vi "Process.vi"(8 "error in (no error)":errorcluster, 11 "RemoteControl":refnum<class "RemoteControl.lvclass">) -> (0 "error out":errorcluster, 3 "RemoteControl out":refnum<class "RemoteControl.lvclass">)   [LabVIEW 2019, in "RemoteControl.lvlib" / "RemoteControl.lvclass"]
doc: "---------------------------------------------------------------\nJKI State Machine Objects™\nhttp://jki.net/state-machine-objects/\nCopyright (C) 2005-2015, JKI <info@jki.net>\nALL RIGHTS RESERVED"
uses:
  RemoteControl.lvclass
  C:/Program Files/National Instruments/LabVIEW 2019/vi.lib/JKI/JKI SMO/SMO/SMO.lvclass
  RemoteControl.lvclass/RemoteControl.ctl
  Typedefs/Message--Cluster.ctl
  <vilib>/JKI/JKI SMO/SMO/Typedefs/Public Events.ctl
  <vilib>/JKI/JKI SMO/SMO/Typedefs/SMOState --Enum.ctl
  <vilib>/JKI/JKI SMO/SMO/Typedefs/Reserve State--Enum.ctl
  <vilib>/JKI/JKI SMO/SMO/SMO.lvclass/SMO.ctl
  Typedefs/RC Process Type--Enum.ctl
  <vilib>/JKI/JKI SMO/SMO/Private/ReftoDVR--SMO.vi
  <vilib>/dlg_ctls.llb/Space Constant.vi
  <vilib>/AdvancedString/1D String Array to Delimited String.vi
  <vilib>/JKI/JKI SMO/SMO/SMO.lvclass
  <userlib>/LevyLab/Debug/Debug.lvlib
panel:
  in  "create message error":bool
  out "Process Type":string
  out "Message Out":string
  out "Message In":string
  in  "delay response":bool
  in  "create server error":bool
  in  "create listener error":bool
  out "State History":string
  out "Connections":i32
  in  "Message Timing?":bool
  in  "timeout (ms)":i32=500
  in  "stop":bool
  # "Remote Control"
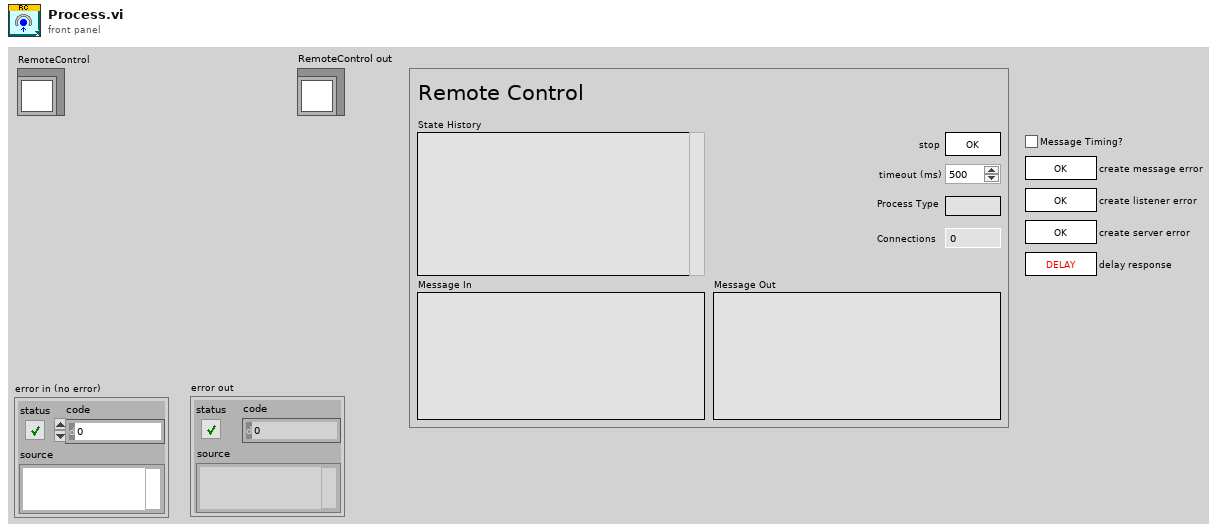
[diagram p1: front panel]
types:
  T1 = enum32{"invalid app kind", "Development System", "Run Time System", "Student Edition", "Embedded LabVIEW", "Evaluation", "Custom"}
  T2 = enum32{"Invalid", "Standard", "Closed", "Hidden", "Minimized", "Maximized"}
  T3 = typedef "RemoteControl.lvlib/RemoteControl.lvclass/Message--Cluster.ctl" = cluster{"Command":string, "Data":variant, "ID":string, "error":errorcluster}
  T4 = typedef "RemoteControl.lvlib/RemoteControl.lvclass/RC Process Type--Enum.ctl" = enum16{"Listener", "Server", "Client"}
  T5 = typedef "RemoteControl.lvlib/RemoteControl.lvclass/PrivateEvents--RemoteControl.Configure.ctl" = cluster{"address":string, "Port":u16, "AllowedRemote":string, "Commands":string[], "timeout":i32}
  T6 = cluster{"Core":cluster{"Current VI Reference":refnum<vi>, "Close Panel on Exit?":bool, "Last Error":cluster{"error":errorcluster, "previous state":string, "remaining states":string}, "Shutdown?":bool}, "SMO":refnum<class "RemoteControl.lvclass">, "Listener":refnum<class "RemoteControl.lvclass">, "RC Process Type":T4, "Configure":T5, "Messages (in)":T3[], "Messages (out)":T3[], "state":enum16{"waiting", "processing"}, "to":i32}
  T7 = cluster{"Current VI Reference":refnum<vi>, "Close Panel on Exit?":bool, "Last Error":cluster{"error":errorcluster, "previous state":string, "remaining states":string}, "Shutdown?":bool}
  T8 = typedef "Debug.lvlib/Attribute.Debug.lvclass/DebugBehavior.ctl" = enum16{"Normal", "Debug"}
  T9 = typedef "SMO.lvclass/Public Events.ctl" = cluster{"Error":refnum<user-event>, "State":refnum<user-event>, "Reserve State":refnum<user-event>}
  T10 = typedef "SMO.lvclass/Protected Events.ctl" = cluster{"StopProcesses":refnum<user-event>, "AbortProcesses":refnum<user-event>, "Config Changed":refnum<user-event>, "Dependency":refnum<user-event>}
  T11 = typedef "RemoteControl.lvlib/RemoteControl.lvclass/PrivateEvents--Cluster.ctl" = cluster{"Configure":refnum<user-event>, "SendMessageToProcess":refnum<user-event>}
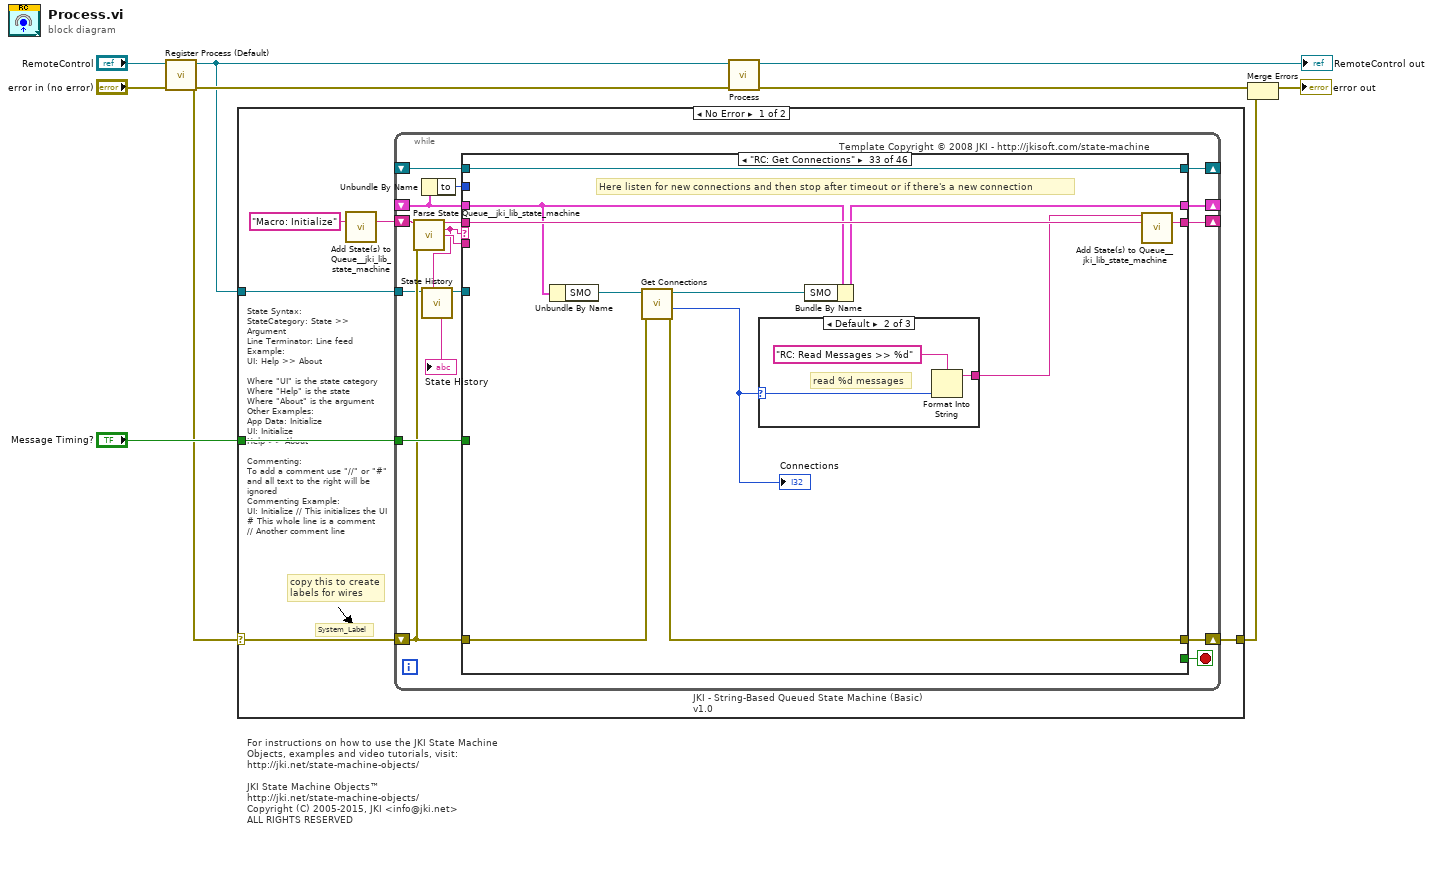
[diagram p0: block diagram]
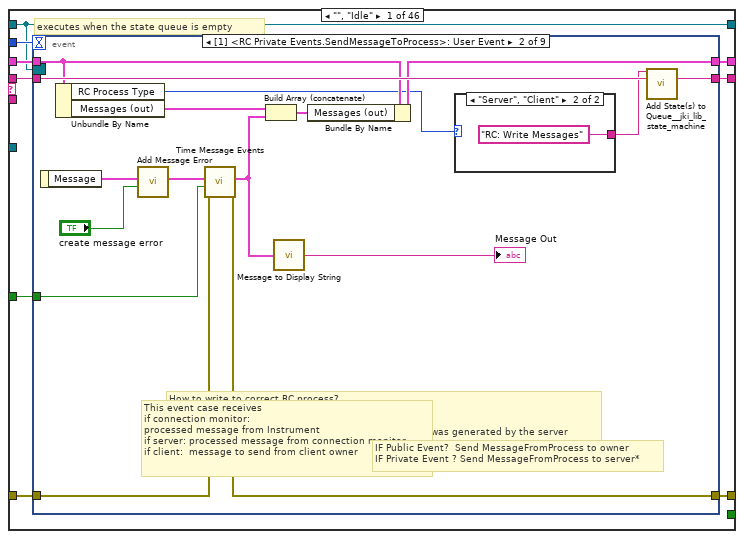
[diagram p2: hidden frame]
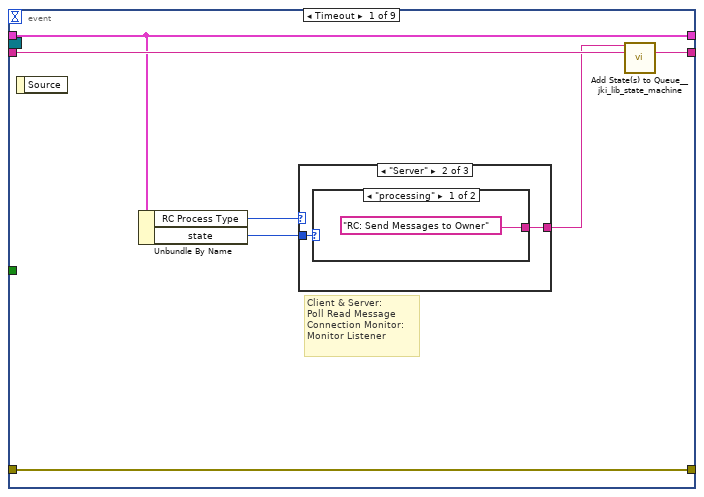
[diagram p3: hidden frame]
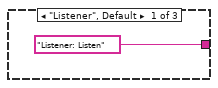
[diagram p4: hidden frame]
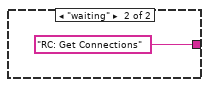
[diagram p5: hidden frame]
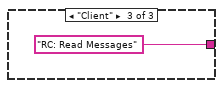
[diagram p6: hidden frame]
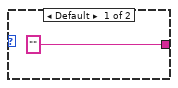
[diagram p7: hidden frame]
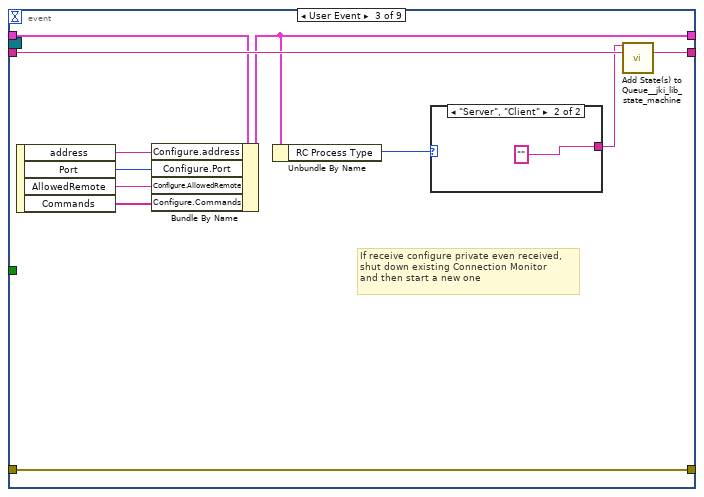
[diagram p8: hidden frame]
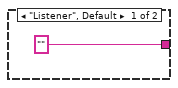
[diagram p9: hidden frame]
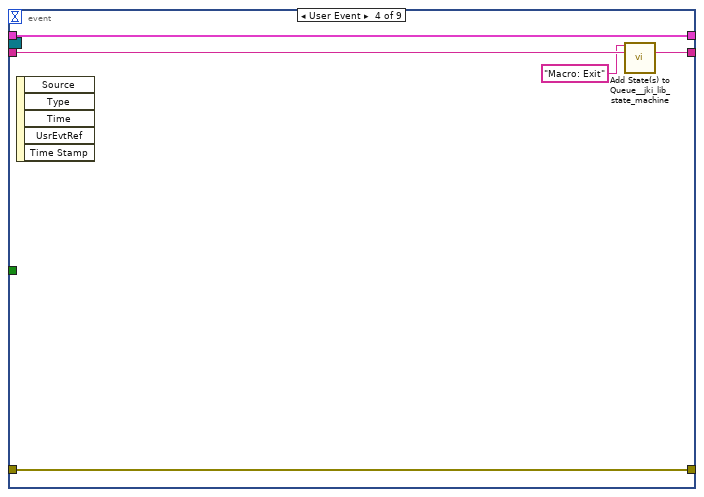
[diagram p10: hidden frame]
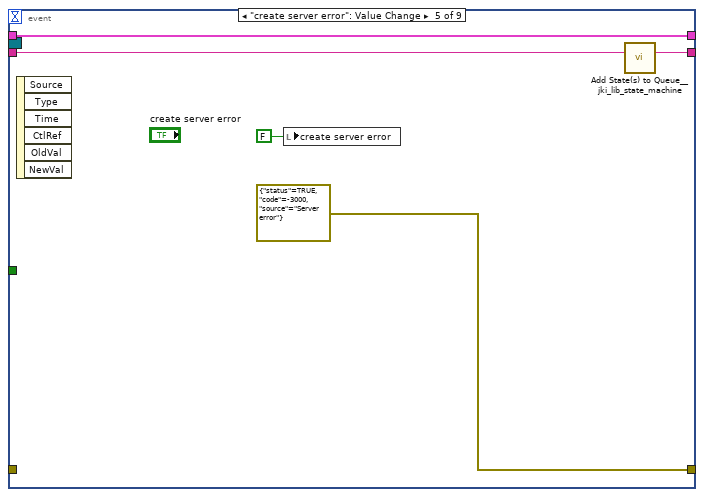
[diagram p11: hidden frame]
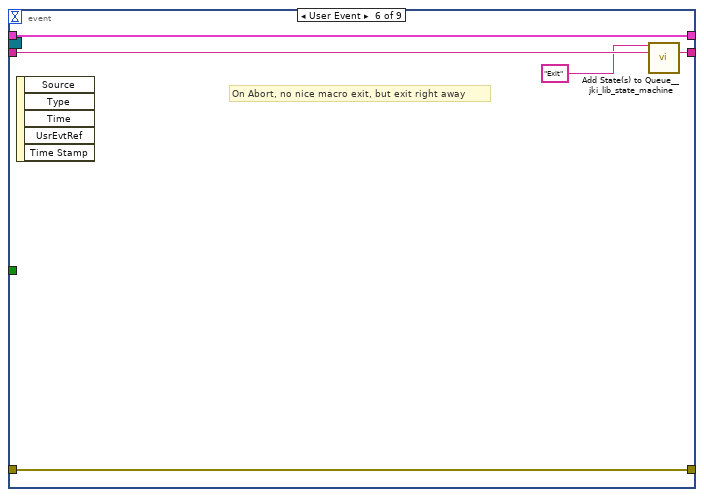
[diagram p12: hidden frame]
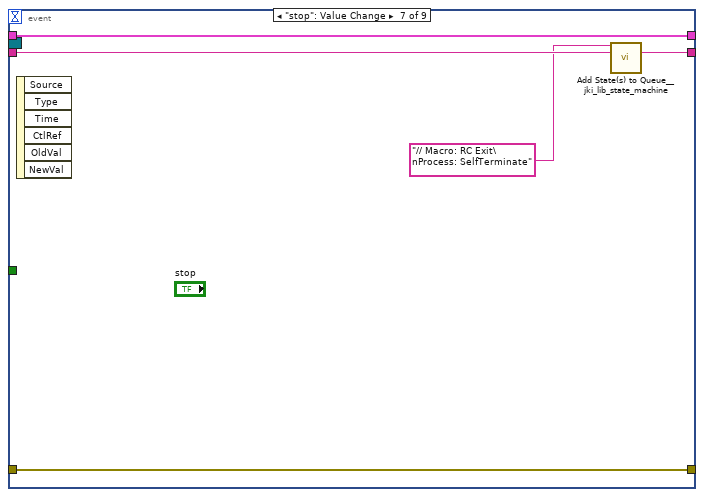
[diagram p13: hidden frame]
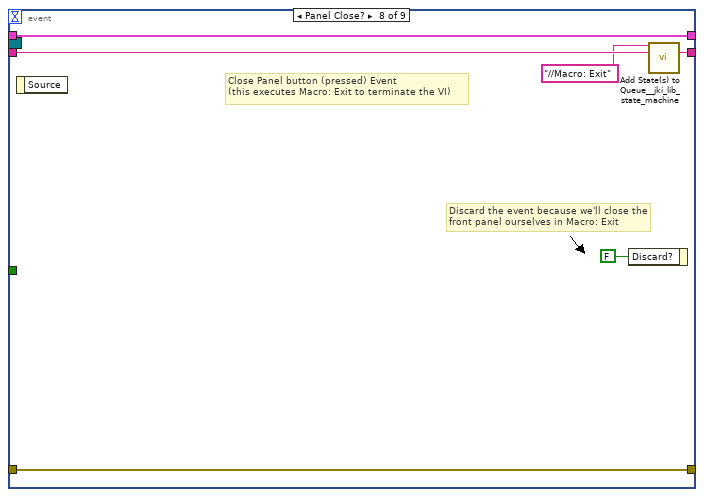
[diagram p14: hidden frame]
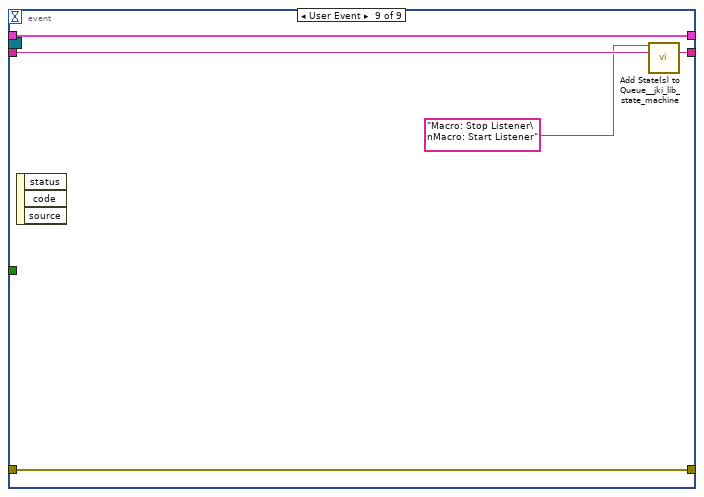
[diagram p15: hidden frame]
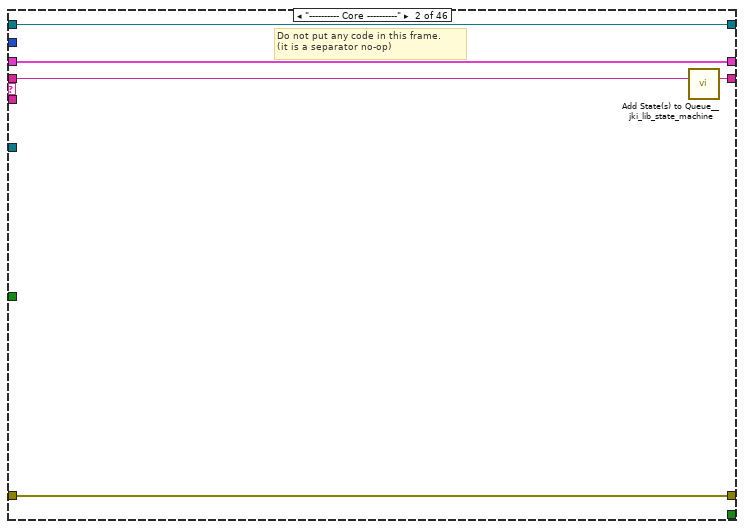
[diagram p16: hidden frame]
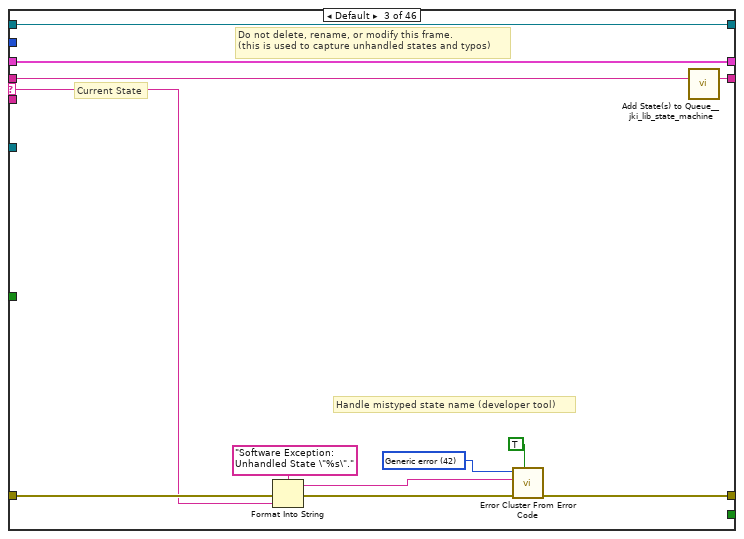
[diagram p17: hidden frame]
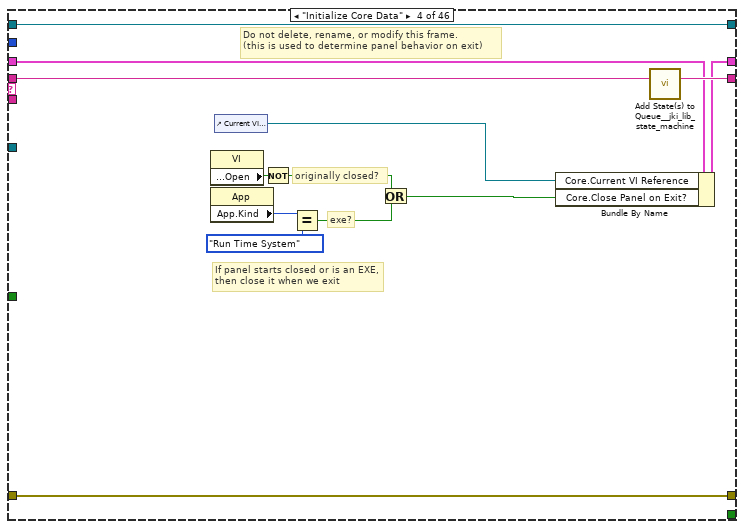
[diagram p18: hidden frame]
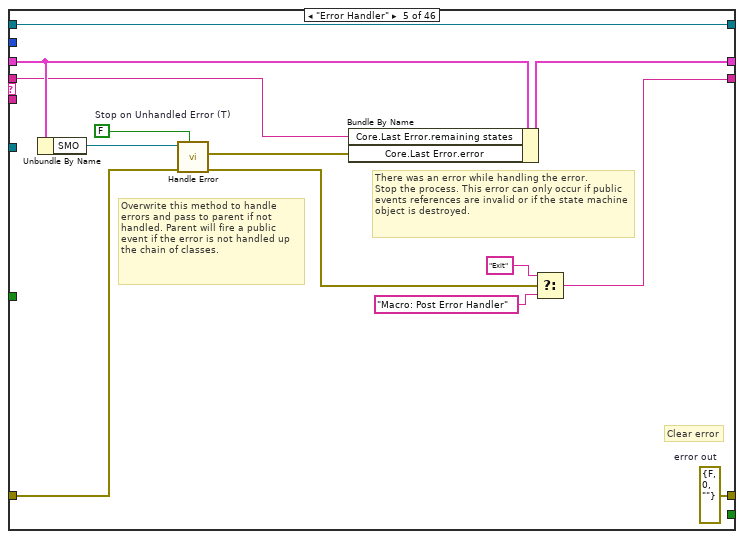
[diagram p19: hidden frame]
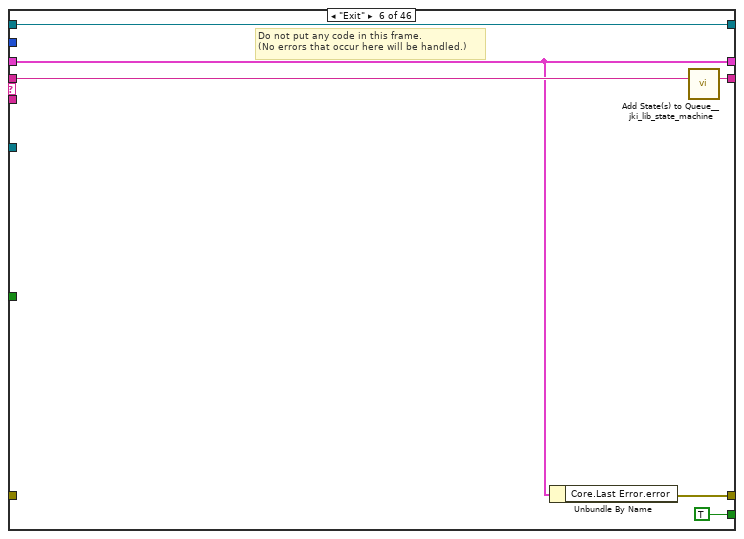
[diagram p20: hidden frame]
diagram:
  # "For instructions on how to use the JKI State Machine Objects, examples and video tutorials, visit:\nhttp://jki.net/state-machine-objects/\n\nJKI State Machine Objects™\nhttp://jki.net/state-machine-objects/\nCopyright (C) 2005-2015, JKI <info@jki.net>\nALL RIGHTS RESERVED"
  n1 = call <vilib>:"Register Process (Default).vi"("error in (no error)"="error in (no error)", "SMO"="RemoteControl") -> ("error out"=w3:errorcluster, "SelfRef"=w2:refnum<class "RemoteControl.lvclass">)  [unwired: 8 in]
  n2 = case shown="No Error" w3 {
    selector: w3 -> [w12 w656]
    tunnel: w2 -> [w13 _]
    tunnel: [w11 w656] -> w5
    tunnel: "Message Timing?" -> [w10 _]
    frame No Error {
      # "State Syntax:\nStateCategory: State >> Argument\nLine Terminator: Line feed\nExample:\nUI: Help >> About\n\nWhere \"UI\" is the state category\nWhere \"Help\" is the state\nWhere \"About\" is the argument\nOther Examples:\nApp Data: Initialize\nUI: Initialize\nHelp >> About\n\nCommenting:\nTo add a comment use \"//\" or \"#\" and all text to the right will be ignored\nCommenting Example:\nUI: Initialize // This initializes the UI\n# This whole line is a comment\n// Another comment line"
      # "copy this to create labels for wires"
      # "System_Label"
      n3 = call <vilib>:"Add State(s) to Queue__jki_lib_state_machine.vi"("State(s) in (\"\")"="Macro: Initialize") -> ("States Out"=w15:string)  [unwired: 14 in]
      n4 = while "JKI - String-Based Queued State Machine (Basic) v1.0" {
        shift-right: [w27] -> _
        shift-left: _ -> [w20]
        shift-right: [w29] -> w11
        shift-left: w12 -> [w23]
        shift-right: [w21] -> _
        shift-left: w15 -> [w30]
        tunnel: w13 -> [w16]
        shift-right: [w26] -> _
        shift-left: _ -> [w25]
        tunnel: w10 -> [w24]
        stop <- w28 stop-if-true
        # "Template Copyright © 2008 JKI - http://jkisoft.com/state-machine"
        n5 = call <vilib>:"Parse State Queue__jki_lib_state_machine.vi"("State Queue"=w30, "Error In (no error)"=w23) -> ("Remaining States"=w32:string, "Current State"=w22:string, "Arguments"=w31:string)  [unwired: 11 in]
        n6 = Unbundle By Name(w20) -> ("to"=w19:i32)
        n7 = call <userlib>:"State History.vi"("Current State"=w22, "SMO"=w16) -> ("SMO"=w17:refnum<class "RemoteControl.lvclass">, "History"=→"State History":string)  [unwired: 8 in]
        n8 = case shown="\"RC: Get Connections\"" w22 {
          selector: w22 -> [_ _ w123 _ _ _ _ _ _ _ _ _ _ _ _ _ _ _ _ _ _ _ _ _ _ _ _ _ _ _ _ _ _ _ _ _ _ _ _ _ _ _ _ _ _ _]
          tunnel: w32 -> [w41 w121 w127 w146 w149 w165 w170 w185 w192 w197 w207 w218 w234 w269 w274 w286 w301 w314 w326 w337 w346 w363 w385 w390 w401 w410 w415 w429 w443 w449 w454 w463 w482 w509 w538 w559 w572 w581 w590 w597 w608 w619 w624 w633 w645 w655]
          tunnel: w31 -> [_ _ _ _ _ _ _ _ _ _ _ w212 w229 w263 _ _ _ _ _ _ _ _ _ _ _ _ _ _ _ _ _ _ _ _ _ _ _ _ _ _ _ _ _ _ _ _]
          tunnel: [w38 w119 w129 w143 w158 w160 w168 w177 w189 w195 w199 w213 w227 w264 w272 w284 w292 w310 w318 w329 w344 w361 w383 w388 w393 w403 w413 w423 w438 w445 w450 w460 w472 w502 w531 w551 w567 w573 w582 w591 w603 w614 w620 w628 w634 w650] -> w29
          tunnel: [w40 w120 w126 w145 w152 w164 w169 w184 w191 w196 w206 w217 w233 w268 w273 w285 w300 w313 w325 w336 w345 w362 w384 w389 w400 w409 w414 w428 w442 w448 w453 w462 w481 w508 w537 w558 w571 w580 w589 w596 w607 w618 w623 w632 w644 w654] -> w21
          tunnel: [_ _ _ _ _ TRUE _ _ _ _ _ _ _ _ _ _ _ _ _ _ _ _ _ _ _ _ _ _ _ _ _ _ _ _ _ _ _ _ _ _ _ _ _ _ _ _] -> w28
          tunnel: [w36 w118 w125 w144 w156 w161 w167 w181 w188 w194 w204 w216 w231 w266 w271 w276 w290 w308 w322 w333 w341 w359 w374 w387 w398 w407 w412 w427 w441 w447 w452 w455 w479 w505 w529 w554 w568 w577 w584 w592 w600 w612 w622 w626 w641 w649] -> w27
          tunnel: w19 -> [w35 _ _ _ _ _ _ _ _ _ _ _ _ _ _ _ _ _ _ _ _ _ _ _ _ _ _ _ _ _ _ _ _ _ _ _ _ _ _ _ _ _ _ _ _ _]
          tunnel: w17 -> [_ _ _ _ _ _ _ w173 _ _ _ _ _ _ _ _ _ _ _ _ _ _ _ _ _ _ _ _ _ _ _ _ _ _ _ _ _ _ _ _ _ _ _ _ _ _]
          tunnel: [w34 w117 w122 w134 w159 w162 w166 w183 w187 w193 w205 w215 w228 w267 w270 w283 w299 w312 w324 w335 w343 w360 w379 w386 w399 w408 w411 w426 w440 w446 w451 w461 w480 w507 w536 w557 w570 w579 w588 w595 w606 w617 w621 w631 w643 w653] -> w26
          tunnel: w25 -> [w34 w117 w122 w134 w159 w162 w166 w183 w187 w193 w205 w215 w228 w267 w270 w283 w299 w312 w324 w335 w343 w360 w379 w386 w399 w408 w411 _ w436 w446 w451 w461 w480 w507 w536 w557 w570 w579 w588 w595 w606 w617 w621 w631 w643 w653]
          tunnel: w24 -> [w33 _ _ _ _ _ _ _ _ _ _ _ _ _ _ _ _ _ _ _ _ _ _ _ _ _ _ _ _ _ _ w458 _ w506 w534 _ _ _ _ _ _ _ _ _ _ _]
          tunnel: w23 -> [w37 w119 w128 w143 w154 _ w168 w177 w190 w195 w198 w214 w232 w265 w272 w284 w291 w310 w319 w330 w344 w361 w383 w388 w394 w404 w413 w424 w439 w445 w450 w457 w476 w495 w532 w552 w560 w574 w583 w594 w604 w615 w620 w629 w638 w651]
          tunnel: w20 -> [w39 w118 w125 w137 w157 w161 w167 _ w188 w194 w204 w216 w231 w266 w271 w276 w289 w308 w322 w333 w341 w356 w373 w387 w398 w402 w412 w427 w441 w447 w452 w455 w478 w497 w530 w555 w569 w578 w585 w592 w601 w609 w622 w625 w642 w649]
          frame "", "Idle" {
            # "executes when the state queue is empty"
            n9 = event shown="[1] <RC Private Events.SendMessageToProcess>: User Event" {
              selector: w34 -> [_ _ _ _ _ _ _ _ _]
              dyn-events: _ -> [_ _ _ _ _ _ _ _ _]
              timeout: w35 -> [_ _ _ _ _ _ _ _ _]
              tunnel: w41 -> [w48 w70 w82 w90 w95 w100 w104 w111 w116]
              tunnel: [w47 w69 w81 w89 w94 w99 w105 w110 w115] -> w40
              tunnel: w39 -> [w43 w66 w80 w87 w93 w97 w103 w108 w113]
              tunnel: [w46 w63 w83 w88 errorcluster {"status"=TRUE, "code"=-3000, "source"="Server error"} ("t") w98 w101 w109 w114] -> w38
              tunnel: w37 -> [w46 w62 w83 w88 _ w98 w101 w109 w114]
              tunnel: [w43 w68 w78 w87 w93 w97 w103 w108 w113] -> w36
              tunnel: w33 -> [_ w58 _ _ _ _ _ _ _]
              event Timeout {
                # "Client & Server:\nPoll Read Message\nConnection Monitor:\nMonitor Listener"
                n10 = event-data() -> ()  [unwired: 1 in, 1 out]
                n11 = Unbundle By Name(w43) -> ("RC Process Type"=w44:T4, "state"=w42:enum16{"waiting", "processing"})
                n12 = case shown="\"Server\"" w44 {
                  tunnel: ["Listener: Listen" ("State(s) in Front (\"\")") w51 "RC: Read Messages" ("State(s) in Front (\"\")")] -> w45
                  tunnel: w42 -> [_ w50 _]
                  frame "Listener", Default {
                  }
                  frame "Server" {
                    n13 = case shown="\"processing\"" w50 {
                      tunnel: ["RC: Send Messages to Owner" ("State(s) in Front (\"\")") "RC: Get Connections" ("State(s) in Front (\"\")")] -> w51
                      frame "processing" {
                      }
                      frame "waiting" {
                      }
                    }
                  }
                  frame "Client" {
                  }
                }
                n14 = call <vilib>:"Add State(s) to Queue__jki_lib_state_machine.vi"("State(s) in Front (\"\")"=w45, "State(s) in (\"\")"=w48) -> ("States Out"=w47:string)  [unwired: 13 in]
              }
              event User Event {
                # "IF Public Event?  Send MessageFromProcess to owner\nIF Private Event ? Send MessageFromProcess to server*"
                # "How to write to correct RC process?\nsomehow keep track of elements in\nserver SMO array\nMessage ID was generated when original public event was generated by the server"
                # "This event case receives\nif connection monitor:\nprocessed message from Instrument\nif server: processed message from connection monitor\nif client:  message to send from client owner"
                n15 = event-data() -> ("Message"=w57:T3)  [unwired: 1 in]
                n16 = Unbundle By Name(w66) -> ("RC Process Type"=w61:T4, "Messages (out)"=w65:T3[])
                n17 = call "Add Message Error.vi"("create message error"="create message error", "Message in"=w57) -> ("Message out"=w56:T3)  [unwired: 9 in]
                n18 = call "Time Message Events.vi"("error in (no error)"=w62, "Debug Mode"=w58, "Message in"=w56) -> ("error out"=w63:errorcluster, "Message out"=w59:T3)  [unwired: 5 in, 2 out]
                n19 = Build Array (concatenate)(w65, w59) -> (w64:T3[])
                n20 = call "Message to Display String.vi"("Message"=w59) -> ("message string"=→"Message Out":string)
                n21 = Bundle By Name(cluster=w66, "Messages (out)"=w64) -> (w68:T6)
                n22 = case shown="\"Server\", \"Client\"" w61 {
                  tunnel: ["" ("State(s) in Front (\"\")") "RC: Write Messages" ("State(s) in Front (\"\")")] -> w67
                  frame Default {
                  }
                  frame "Server", "Client" {
                  }
                }
                n23 = call <vilib>:"Add State(s) to Queue__jki_lib_state_machine.vi"("State(s) in Front (\"\")"=w67, "State(s) in (\"\")"=w70) -> ("States Out"=w69:string)  [unwired: 13 in]
              }
              event User Event {
                # "If receive configure private even received,\nshut down existing Connection Monitor \nand then start a new one"
                n24 = event-data() -> ("address"=w73:string, "Port"=w74:u16, "AllowedRemote"=w75:string, "Commands"=w76:string[])  [unwired: 1 in]
                n25 = Bundle By Name(cluster=w80, "Configure.address"=w73, "Configure.Port"=w74, "Configure.AllowedRemote"=w75, "Configure.Commands"=w76) -> (w78:T6)
                n26 = Unbundle By Name(w78) -> ("RC Process Type"=w79:T4)
                n27 = case shown="\"Server\", \"Client\"" w79 {
                  tunnel: ["" ("State(s) in Front (\"\")") "" ("State(s) in Front (\"\")")] -> w77
                  frame "Listener", Default {
                  }
                  frame "Server", "Client" {
                  }
                }
                n28 = call <vilib>:"Add State(s) to Queue__jki_lib_state_machine.vi"("State(s) in Front (\"\")"=w77, "State(s) in (\"\")"=w82) -> ("States Out"=w81:string)  [unwired: 13 in]
              }
              event User Event {
                n29 = event-data() -> ()  [unwired: 1 in, 5 out]
                n30 = call <vilib>:"Add State(s) to Queue__jki_lib_state_machine.vi"("State(s) in Front (\"\")"="Macro: Exit", "State(s) in (\"\")"=w90) -> ("States Out"=w89:string)  [unwired: 13 in]
              }
              event "create server error": Value Change {
                n31 = event-data() -> ()  [unwired: 1 in, 6 out]
                n32 = local write "create server error"(FALSE ("create listener error")) -> ()
                n33 = call <vilib>:"Add State(s) to Queue__jki_lib_state_machine.vi"("State(s) in (\"\")"=w95) -> ("States Out"=w94:string)  [unwired: 14 in]
              }
              event User Event {
                # "On Abort, no nice macro exit, but exit right away"
                n34 = event-data() -> ()  [unwired: 1 in, 5 out]
                n35 = call <vilib>:"Add State(s) to Queue__jki_lib_state_machine.vi"("State(s) in Front (\"\")"="Exit", "State(s) in (\"\")"=w100) -> ("States Out"=w99:string)  [unwired: 13 in]
              }
              event "stop": Value Change {
                n36 = event-data() -> ()  [unwired: 1 in, 6 out]
                n37 = call <vilib>:"Add State(s) to Queue__jki_lib_state_machine.vi"("State(s) in Front (\"\")"="// Macro: RC Exit\nProcess: SelfTerminate" ("State(s) in Front (\"\")"), "State(s) in (\"\")"=w104) -> ("States Out"=w105:string)  [unwired: 13 in]
              }
              event Panel Close? {
                # "Discard the event because we'll close the front panel ourselves in Macro: Exit"
                # "Close Panel button (pressed) Event\n(this executes Macro: Exit to terminate the VI)"
                n38 = event-data() -> ()  [unwired: 1 in, 1 out]
                n39 = event-data("Discard?"=FALSE) -> ()  [unwired: 1 in, 1 out]
                n40 = call <vilib>:"Add State(s) to Queue__jki_lib_state_machine.vi"("State(s) in Front (\"\")"="//Macro: Exit", "State(s) in (\"\")"=w111) -> ("States Out"=w110:string)  [unwired: 13 in]
              }
              event User Event {
                n41 = event-data() -> ()  [unwired: 1 in, 3 out]
                n42 = call <vilib>:"Add State(s) to Queue__jki_lib_state_machine.vi"("State(s) in Front (\"\")"="Macro: Stop Listener\nMacro: Start Listener", "State(s) in (\"\")"=w116) -> ("States Out"=w115:string)  [unwired: 13 in]
              }
            }
          }
          frame "---------- Core ----------" {
            # "Do not put any code in this frame.\n(it is a separator no-op)"
            n43 = call <vilib>:"Add State(s) to Queue__jki_lib_state_machine.vi"("State(s) in (\"\")"=w121) -> ("States Out"=w120:string)  [unwired: 14 in]
          }
          frame Default {
            w132 = 42 items=["No error", "Argument error", "Memory is full", "Out of zone", "End of file", "File already open", "Generic file I/O error", "File not found", "File permission error", "Disk is full", "Duplicate path", "Too many files open", "System feature not enabled", "Resource file not found", "Cannot add resource", "Resource not found", "Image not found", "Image memory error", "Pen does not exist", "Config type invalid", "Config token not found", "Config parse error", "Config memory error", "Bad external code format", "Bad external code offset", "External code not present", "Null window", "Destroy window error", "Null menu", "Print aborted", "Bad print record", "Print driver error", "Windows error during printing", "Memory error during printing", "Print dialog error", "Generic print error", "Invalid device refnum", "Device not found", "Device parameter error", "Device unit error", "Cannot open device", "Device call aborted", "Generic error", "Cancelled by user", "Object ID too low", "Object ID too high", "Object not in heap", "Unknown heap", "Unknown object (invalid DefProc)", "Unknown object (DefProc not in table)", "Message out of range", "Invalid (null) method", "Unknown message", "Manager call not supported", "Bad address", "Network operation in progress", "Network operation timed out", "Connection is busy", "Network attribute not supported", "Network error", "Address in use", "System out of memory", "Connection aborted", "Connection refused", "Not connected", "Already connected", "Connection closed", "Initialization error (interapplication manager)", "Bad occurrence", "Wait on unbound occurrence handler", "Occurrence queue overflow", "Datalog type conflict", "Unused", "Unrecognized type (interapplication manager)", "Memory corrupt", "Failed to make temporary DLL", "Old CIN version", "Drag socket not found", "Failed to load drop-object", "Failed to register OLE object", "Failed to release OLE object", "Format specifier type mismatch", "Unknown format specifier", "Too few format specifiers", "Too many format specifiers", "Scan failed", "Newer CIN version", "Error converting to variant", "Runtime menu error", "Password tampered", "Variant attribute not found", "Incompatible variant data type", "Event data is not available", "Event Store is not present", "Occurrence is not found", "Event Queue is not created", "Event info is not available", "Refnum passed is NULL", "Error retrieving Class GUID", "Error retrieving CoClass GUID", "Error retrieving TypeLib GUID.", "Bad built application magic bytes.", "Specific driver is different from the specific driver associated with the Logical Name.", "There is no session opened to the class driver.", "Max Error", "MAX - Error with config objects", "MAX - Error loading configuration", "MAX - Group not supported"]
            # "Current State"
            # "Do not delete, rename, or modify this frame.\n(this is used to capture unhandled states and typos)"
            # "Handle mistyped state name (developer tool)"
            n44 = Format Into String(format string="Software Exception: Unhandled State \"%s\"." ("message"), error in=w128, w123) -> (resulting string=w131:string, error out=w130:errorcluster)  [unwired: 1 in]
            n45 = call <vilib>:"Error Cluster From Error Code.vi"("show call chain? (False)"=TRUE, "error in (no error)"=w130, "error message (\"\")"=w131, "error code (0)"=w132) -> ("error out"=w129:errorcluster)  [unwired: 5 in]
            n46 = call <vilib>:"Add State(s) to Queue__jki_lib_state_machine.vi"("State(s) in (\"\")"=w127) -> ("States Out"=w126:string)  [unwired: 14 in]
          }
          frame "Initialize Core Data" {
            # "Do not delete, rename, or modify this frame.\n(this is used to determine panel behavior on exit)"
            # "originally closed?"
            # "exe?"
            # "If panel starts closed or is an EXE, then close it when we exit"
            n47 = property class="VI"() -> ("Front Panel.Open"=w142:bool)  [unwired: 2 in, 2 out]
            n48 = property class="App"() -> ("App.Kind"=w141:T1)  [unwired: 2 in, 2 out]
            n49 = control-ref of="Current VI Reference"() -> (w135:refnum<vi>)
            n50 = Not(x=w142) -> (.not. x?=w139:bool)
            n51 = Equal?(x=w141, y=T1."Run Time System" ("Application:Kind")) -> (x = y?=w138:bool)
            n52 = Or(x=w139, y=w138) -> (x .or. y?=w136:bool)
            n53 = Bundle By Name(cluster=w137, "Core.Current VI Reference"=w135, "Core.Close Panel on Exit?"=w136) -> (w144:T6)
            n54 = call <vilib>:"Add State(s) to Queue__jki_lib_state_machine.vi"("State(s) in (\"\")"=w146) -> ("States Out"=w145:string)  [unwired: 14 in]
          }
          frame "Error Handler" {
            w155 = FALSE  # Stop on Unhandled Error (T)
            w158 = errorcluster {"status"=FALSE, "code"=0, "source"=""}  # error out
            # "There was an error while handling the error.\nStop the process. This error can only occur if public events references are invalid or if the state machine object is destroyed."
            # "Clear error"
            # "Overwrite this method to handle errors and pass to parent if not handled. Parent will fire a public event if the error is not handled up the chain of classes."
            n55 = Unbundle By Name(w157) -> ("SMO"=w153:refnum<class "RemoteControl.lvclass">)
            n56 = call-dynamic "Handle Error.vi"("Stop on Unhandled Error (T)"=w155, "error in"=w154, "SMO"=w153) -> ("handling error"=w150:errorcluster, "Unhandled error"=w151:errorcluster)  [unwired: 6 in, 1 out]
            n57 = Bundle By Name(cluster=w157, "Core.Last Error.remaining states"=w149, "Core.Last Error.error"=w151) -> (w156:T6)
            n58 = Select(t="Exit", s=w150, f="Macro: Post Error Handler") -> (s? t:f=w152:string)
          }
          frame "Exit" {
            # "Do not put any code in this frame.\n(No errors that occur here will be handled.)"
            n59 = Unbundle By Name(w161) -> ("Core.Last Error.error"=w160:errorcluster)
            n60 = call <vilib>:"Add State(s) to Queue__jki_lib_state_machine.vi"("State(s) in (\"\")"=w165) -> ("States Out"=w164:string)  [unwired: 14 in]
          }
          frame "---------- Data ----------" {
            # "Do not put any code in this frame.\n(It is a separator no-op. You can make a copy of this frame to create a new Data frame)"
            n61 = call <vilib>:"Add State(s) to Queue__jki_lib_state_machine.vi"("State(s) in (\"\")"=w170) -> ("States Out"=w169:string)  [unwired: 14 in]
          }
          frame "Data: Initialize" {
            w174 = 10  # to
            w175 = enum16{"waiting", "processing"}."waiting"  # state
            w176 = refnum<class "RemoteControl.lvclass"> refnum  # Listener
            w178 = T3[] []  # Messages (out)
            w179 = T3[] []  # Messages (in)
            w182 = T7 {"Current VI Reference"=refnum, "Close Panel on Exit?"=FALSE, "Last Error"={"error"={"status"=FALSE, "code"=0, "source"=""}, "previous state"="", "remaining states"=""}, "Shutdown?"=FALSE}  # Core
            # "do not delete - used by framework"
            # "Initialize the shift-register data, here.\n(data names are defined by what you wire into the bundle function)"
            n62 = Unbundle By Name(w173) -> ("RC Process Type"=w171:T4, "Configure"=w180:T5)
            n63 = Format Into String(w171) -> (resulting string=→"Process Type":string)  [unwired: 3 in, 1 out]
            n64 = Bundle("Core"=w182, "SMO"=w173, "Listener"=w176, "RC Process Type"=w171, "Configure"=w180, "Messages (in)"=w179, "Messages (out)"=w178, "state"=w175, "to"=w174) -> (w181:T6)  [unwired: 1 in]
            n65 = call <vilib>:"Add State(s) to Queue__jki_lib_state_machine.vi"("State(s) in (\"\")"=w185) -> ("States Out"=w184:string)  [unwired: 14 in]
          }
          frame "Data: Cleanup" {
            # "Cleanup any data and references, here.\n(this is called automatically, by the Macro: Exit)"
            n66 = Unbundle By Name(w188) -> ("Core.Current VI Reference"=w186:refnum<vi>)
            n67 = Close Reference(reference=w186, error in (no error)=w190) -> (error out=w189:errorcluster)
            n68 = call <vilib>:"Add State(s) to Queue__jki_lib_state_machine.vi"("State(s) in (\"\")"=w192) -> ("States Out"=w191:string)  [unwired: 14 in]
          }
          frame "---------- UI ----------" {
            # "Do not put any code in this frame.\n(It is a separator no-op. You can make a copy of this frame to create a new UI frame)"
            n69 = call <vilib>:"Add State(s) to Queue__jki_lib_state_machine.vi"("State(s) in (\"\")"=w197) -> ("States Out"=w196:string)  [unwired: 14 in]
          }
          frame "UI: Initialize" {
            # "Initialize the User Interface, here.\n(this is called automatically, by the Macro: Init)"
            n70 = Unbundle By Name(w204) -> ("RC Process Type"=w203:T4)
            n71 = case shown="\"Server\", Default" w203 {
              tunnel: [FALSE TRUE] -> w202
              tunnel: [TRUE FALSE] -> w201
              frame "Listener" {
              }
              frame "Server", Default {
              }
            }
            n72 = call <userlib>:"Fit VI window to Largest Dec__ogtk.vi"("error in (no error)"=w198, "border spacing (2 px)"=0) -> ("error out"=w199:errorcluster)  [unwired: 4 in, 1 out]
            n73 = property on="create server error" class="Bool (strict)"("Visible"=w202) -> ()  [unwired: 2 in, 2 out]
            n74 = property on="create listener error" class="Bool (strict)"("Visible"=w201) -> ()  [unwired: 2 in, 2 out]
            n75 = call <vilib>:"Add State(s) to Queue__jki_lib_state_machine.vi"("State(s) in (\"\")"=w207) -> ("States Out"=w206:string)  [unwired: 14 in]
          }
          frame "UI: Cursor Set" {
            # "Argument"
            # "Initialize the User Interface, here.\n(this is called automatically, by the Macro: Init)"
            n76 = disable-structure shown="Default" {
              disable-tunnel: w214 -> [w219 w222]
              disable-tunnel: [w219 w221] -> w213
              disable-tunnel: w212 -> [_ w220]
              frame condition #0 {
              }
              frame condition #1 (active) {
                n77 = case shown="\"Idle\", Default" w220 {
                  tunnel: w222 -> [w224 w226]
                  tunnel: [w223 w225] -> w221
                  frame "Idle", Default {
                    n78 = call <vilib>:"Unset Busy.vi"("error in (no error)"=w224) -> ("error out"=w223:errorcluster)  [unwired: 10 in]
                  }
                  frame "Busy" {
                    n79 = call <vilib>:"Set Busy.vi"("error in (no error)"=w226) -> ("error out"=w225:errorcluster)  [unwired: 9 in, 1 out]
                  }
                }
              }
            }
            n80 = call <vilib>:"Add State(s) to Queue__jki_lib_state_machine.vi"("State(s) in (\"\")"=w218) -> ("States Out"=w217:string)  [unwired: 14 in]
          }
          frame "UI: Front Panel State" {
            # "Argument"
            # "Set Front Panel Open or Closed\n(Usage: \"UI: Front Panel State >> Open|Close\")"
            n81 = Unbundle By Name(w231) -> ("Core.Current VI Reference"=w230:refnum<vi>)
            n82 = disable-structure shown="Default" {
              disable-tunnel: w232 -> [w238 w259]
              disable-tunnel: [w237 w259] -> w227
              disable-tunnel: w230 -> [w236 _]
              disable-tunnel: w229 -> [w235 _]
              frame condition #0 (active) {
                n83 = case shown="\"Close\"" w235 {
                  tunnel: w238 -> [w242 w253]
                  tunnel: [w243 w254] -> w237
                  tunnel: w236 -> [_ _]
                  frame "Open", Default {
                    n84 = property class="VI"(error in=w242) -> (reference out=w240:refnum<vi>, error out=w241:errorcluster, "FP.State"=w239:T2)  [unwired: 1 in]
                    n85 = case shown="\"Closed\"" w239 {
                      tunnel: [w246 w249] -> w243
                      tunnel: w241 -> [w245 w249]
                      tunnel: w240 -> [w244 _]
                      frame "Closed" {
                        n86 = invoke class="VI" method="FP.Open"(reference=w244, error in=w245, "Activate"=TRUE, "State"=T2."Standard") -> (error out=w246:errorcluster)  [unwired: 1 in, 4 out]
                      }
                      frame Default {
                      }
                    }
                  }
                  frame "Close" {
                    n87 = property class="VI"(error in=w253) -> (reference out=w251:refnum<vi>, error out=w252:errorcluster, "FP.State"=w250:T2)  [unwired: 1 in]
                    n88 = case shown="Default" w250 {
                      tunnel: [w255 w258] -> w254
                      tunnel: w252 -> [w255 w257]
                      tunnel: w251 -> [_ w256]
                      frame "Invalid", "Closed" {
                      }
                      frame Default {
                        n89 = invoke class="VI" method="FP.Close"(reference=w256, error in=w257) -> (error out=w258:errorcluster)  [unwired: 1 in, 2 out]
                      }
                    }
                  }
                }
              }
              frame condition #1 {
              }
            }
            n90 = call <vilib>:"Add State(s) to Queue__jki_lib_state_machine.vi"("State(s) in (\"\")"=w234) -> ("States Out"=w233:string)  [unwired: 14 in]
          }
          frame "UI: Wait" {
            n91 = Scan From String(format string="%d", input string=w263, default 1=u32 0 ("default value 1")) -> (output 1=w261:u32)  [unwired: 2 in, 3 out]
            n92 = call <userlib>:"Wait (ms)__ogtk.vi"("error in (no error)"=w265, "milliseconds to wait"=w261) -> ("error out"=w264:errorcluster)  [unwired: 8 in, 1 out]
            n93 = call <vilib>:"Add State(s) to Queue__jki_lib_state_machine.vi"("State(s) in (\"\")"=w269) -> ("States Out"=w268:string)  [unwired: 14 in]
          }
          frame "---------- Macro ----------" {
            # "Do not put any code in this frame.\n(It is a separator no-op. You can make a copy of this frame to create a new Macro frame)"
            n94 = call <vilib>:"Add State(s) to Queue__jki_lib_state_machine.vi"("State(s) in (\"\")"=w274) -> ("States Out"=w273:string)  [unwired: 14 in]
          }
          frame "Macro: Initialize" {
            # "Initialization Macro\n(This is called once, when the VI starts)"
            n95 = call <vilib>:"Add State(s) to Queue__jki_lib_state_machine.vi"("State(s) in Front (\"\")"="UI: Initialize", "State(s) in (\"\")"="UI: Front Panel State >> Close", "State(s) at Back (\"\")"="Macro: Debug\nMacro: RC Initialize") -> ("States Out"=w277:string)  [unwired: 12 in]
            n96 = call <vilib>:"Add State(s) to Queue__jki_lib_state_machine.vi"("State(s) in Front (\"\")"="Data: Initialize\nInitialize Core Data\nEvents: Register", "State(s) in (\"\")"="Process: Sync", "State(s) at Back (\"\")"=w277) -> ("States Out"=w281:string)  [unwired: 12 in]
            n97 = call <vilib>:"Add State(s) to Queue__jki_lib_state_machine.vi"("State(s) in Front (\"\")"=w281, "State(s) in (\"\")"=w286) -> ("States Out"=w285:string)  [unwired: 13 in]
          }
          frame "Macro: Debug" {
            # "exe?"
            # "If pane is an EXE, then close it when we exit"
            # "Macro: Debug\n(get debug behavior, determine UI and determine shutdown behavior)"
            n98 = Unbundle By Name(w289) -> ("Core.Close Panel on Exit?"=w293:bool, "SMO"=w298:refnum<class "RemoteControl.lvclass">)
            n99 = property class="App"() -> ("App.Kind"=w296:T1)  [unwired: 2 in, 2 out]
            n100 = Equal?(x=w296, y=T1."Run Time System" ("Application:Kind")) -> (x = y?=w288:bool)
            n101 = call <userlib>:"Get Debug Mode.vi"("error in (no error)"=w291, "SMO"=w298) -> ("error out"=w292:errorcluster, "Behavior"=w297:T8)  [unwired: 7 in, 1 out]
            n102 = case shown="\"Normal\", Default" w297 {
              tunnel: [_ "UI: Front Panel State >> Open\nUI: Wait >> 1000"] -> w287
              tunnel: [w303 w304] -> w294
              tunnel: w293 -> [w303 _]
              tunnel: w288 -> [_ w306]
              frame "Normal", Default {
                w302 = FALSE ("Visible")
                # "respect core.close"
                n103 = property on="create server error" class="Bool (strict)"("Visible"=w302) -> ()  [unwired: 2 in, 2 out]
                n104 = property on="create listener error" class="Bool (strict)"("Visible"=w302) -> ()  [unwired: 2 in, 2 out]
              }
              frame "Debug" {
                # "keep panel open\nunless exe"
                n105 = Or(x=w306, y=FALSE) -> (x .or. y?=w304:bool)
              }
            }
            n106 = Bundle By Name(cluster=w289, "Core.Close Panel on Exit?"=w294) -> (w290:T6)
            n107 = call <vilib>:"Add State(s) to Queue__jki_lib_state_machine.vi"("State(s) in Front (\"\")"=w287, "State(s) in (\"\")"=w301) -> ("States Out"=w300:string)  [unwired: 13 in]
          }
          frame "Macro: RC Initialize" {
            n108 = Unbundle By Name(w308) -> ("RC Process Type"=w311:T4)
            n109 = case shown="\"Server\"" w311 {
              tunnel: ["Listener: Start Listener" ("State(s) in Front (\"\")") "Macro: Start Listener\nRC: Open Server Connection" ("State(s) in Front (\"\")") "RC: Open Client Connection" ("State(s) in Front (\"\")")] -> w309
              frame "Listener", Default {
              }
              frame "Server" {
              }
              frame "Client" {
              }
            }
            n110 = call <vilib>:"Add State(s) to Queue__jki_lib_state_machine.vi"("State(s) in Front (\"\")"=w309, "State(s) in (\"\")"=w314) -> ("States Out"=w313:string)  [unwired: 13 in]
          }
          frame "Macro: Start Listener" {
            n111 = Unbundle By Name(w322) -> ("SMO"=w321:refnum<class "RemoteControl.lvclass">)
            n112 = call <vilib>:"Get LV Class Name.vi"("error in (no error)"=w319, "object"=w321) -> ("error out"=w318:errorcluster, "class name"=w320:string)  [unwired: 8 in]
            n113 = case shown="\"RemoteControl.STM.lvclass\"" w320 {
              tunnel: ["" ("State(s) in Front (\"\")") "RC: Create Listener SMO\nEvents: Register Listener SMO\nRC: Start Listener SMO" ("State(s) in Front (\"\")")] -> w323
              frame Default {
              }
              frame "RemoteControl.STM.lvclass" {
              }
            }
            n114 = call <vilib>:"Add State(s) to Queue__jki_lib_state_machine.vi"("State(s) in Front (\"\")"=w323, "State(s) in (\"\")"=w326) -> ("States Out"=w325:string)  [unwired: 13 in]
          }
          frame "Macro: Stop Listener" {
            n115 = Unbundle By Name(w333) -> ("SMO"=w332:refnum<class "RemoteControl.lvclass">)
            n116 = call <vilib>:"Get LV Class Name.vi"("error in (no error)"=w330, "object"=w332) -> ("error out"=w329:errorcluster, "class name"=w331:string)  [unwired: 8 in]
            n117 = case shown="\"RemoteControl.STM.lvclass\"" w331 {
              tunnel: ["" ("State(s) in Front (\"\")") "RC: Stop Listener SMO\nRC: Destroy Listener SMO" ("State(s) in Front (\"\")")] -> w334
              frame Default {
              }
              frame "RemoteControl.STM.lvclass" {
              }
            }
            n118 = call <vilib>:"Add State(s) to Queue__jki_lib_state_machine.vi"("State(s) in Front (\"\")"=w334, "State(s) in (\"\")"=w337) -> ("States Out"=w336:string)  [unwired: 13 in]
          }
          frame "Macro: RC Exit" {
            n119 = Unbundle By Name(w341) -> ("RC Process Type"=w340:T4)
            n120 = case shown="\"Server\"" w340 {
              tunnel: ["Listener: Stop Listener" ("State(s) in Front (\"\")") "Macro: Stop Listener\nRC: Close Connection" ("State(s) in Front (\"\")")] -> w342
              frame "Listener", Default {
              }
              frame "Server" {
              }
            }
            n121 = call <vilib>:"Add State(s) to Queue__jki_lib_state_machine.vi"("State(s) in Front (\"\")"=w342, "State(s) in (\"\")"=w346) -> ("States Out"=w345:string)  [unwired: 13 in]
          }
          frame "Macro: Post Error Handler" {
            # "Clear Last Error?"
            n122 = Unbundle By Name(w356) -> ("Core.Last Error.error"=w351:errorcluster)
            n123 = Unbundle By Name(w356) -> ("RC Process Type"=w352:T4, "Core.Last Error.remaining states"=w355:string, "Core.Shutdown?"=w354:bool)
            n124 = case shown="False" FALSE {
              tunnel: w351 -> [w364 _]
              tunnel: [w364 _] -> w349
              frame False {
              }
              frame True {
              }
            }
            n125 = case shown="False" w354 {
              tunnel: w355 -> [_ w370]
              tunnel: [w365 w369] -> w353
              tunnel: w352 -> [w366 _]
              frame False {
                # "These are the remaining states (at the moment the error occured). States can be altered according to business logic."
                # "NOT SHUTTING DOWN"
                n126 = case shown="\"Server\"" w366 {
                  tunnel: ["" ("State(s) in Front (\"\")") "Macro: RC Exit\nMacro: RC Initialize" ("State(s) in Front (\"\")")] -> w365
                  frame Default {
                    # "If Listener, owner will restart\nListener process"
                  }
                  frame "Server" {
                  }
                }
              }
              frame True {
                # "Developer can decide to alter the states but should be aware that during the shutdown process, there are certain states that must be run for the SMO to properly shut itself (and this process) down. As such, one can add states to perform additional clean-ups, but should append the remaining state to be executed."
                # "SHUTTING DOWN"
                n127 = call <vilib>:"Add State(s) to Queue__jki_lib_state_machine.vi"("State(s) in (\"\")"=w370) -> ("States Out"=w369:string)  [unwired: 14 in]
              }
            }
            n128 = Bundle By Name(cluster=w356, "Core.Last Error.error"=w349, "Messages (out)"=T3[] [], "state"=enum16{"waiting", "processing"}."waiting") -> (w359:T6)
            n129 = call <vilib>:"Add State(s) to Queue__jki_lib_state_machine.vi"("State(s) in Front (\"\")"=w353, "State(s) in (\"\")"=w363) -> ("States Out"=w362:string)  [unwired: 13 in]
          }
          frame "Macro: Exit" {
            # "Exit Macro\n(This is called once, when the VI exits)"
            n130 = Unbundle By Name(w373) -> ("Core.Close Panel on Exit?"=w375:bool)
            n131 = Bundle By Name(cluster=w373, "Core.Shutdown?"=TRUE) -> (w374:T6)
            n132 = Select(t="UI: Front Panel State >> Close", s=w375, f="") -> (s? t:f=w381:string)
            n133 = call <vilib>:"Add State(s) to Queue__jki_lib_state_machine.vi"("State(s) in Front (\"\")"="Macro: RC Exit", "State(s) at Back (\"\")"="Data: Cleanup\nEvents: Unregister\nProcess: Sync\nExit") -> ("States Out"=w376:string)  [unwired: 13 in]
            n134 = call <vilib>:"Add State(s) to Queue__jki_lib_state_machine.vi"("State(s) in (\"\")"=w381, "State(s) at Back (\"\")"=w376) -> ("States Out"=w380:string)  [unwired: 13 in]
            n135 = call <vilib>:"Add State(s) to Queue__jki_lib_state_machine.vi"("State(s) in Front (\"\")"=w380, "State(s) in (\"\")"=w385) -> ("States Out"=w384:string)  [unwired: 13 in]
          }
          frame "---------- Process ----------" {
            # "Template Separator\n(You can make a copy of, or modify, this frame)"
            n136 = call <vilib>:"Add State(s) to Queue__jki_lib_state_machine.vi"("State(s) in (\"\")"=w390) -> ("States Out"=w389:string)  [unwired: 14 in]
          }
          frame "Process: Sync" {
            n137 = Unbundle By Name(w398) -> ("SMO"=w391:refnum<class "RemoteControl.lvclass">)
            n138 = call <vilib>:"WaitOnProcessSync.vi"("error in (no error)"=w394, "SMO"=w391) -> ("error out"=w393:errorcluster, "Don't run?"=w397:bool)  [unwired: 7 in, 1 out]
            n139 = Select(t="Data: Cleanup\nEvents: Unregister\nExit", s=w397, f="") -> (s? t:f=w392:string)
            n140 = call <vilib>:"Add State(s) to Queue__jki_lib_state_machine.vi"("State(s) in Front (\"\")"=w392, "State(s) in (\"\")"=w401) -> ("States Out"=w400:string)  [unwired: 13 in]
          }
          frame "Process: SelfTerminate" {
            n141 = Unbundle By Name(w402) -> ("SMO"=w406:refnum<class "RemoteControl.lvclass">)
            n142 = call <vilib>:"SelfTerminate.vi"("error in (no error)"=w404, "SMO in"=w406) -> ("error out"=w403:errorcluster, "SMO out"=w405:refnum<class "RemoteControl.lvclass">)  [unwired: 8 in]
            n143 = Bundle By Name(cluster=w402, "SMO"=w405) -> (w407:T6)
            n144 = call <vilib>:"Add State(s) to Queue__jki_lib_state_machine.vi"("State(s) in (\"\")"=w410) -> ("States Out"=w409:string)  [unwired: 14 in]
          }
          frame "---------- Events ----------" {
            # "Template Separator\n(You can make a copy of, or modify, this frame)"
            n145 = call <vilib>:"Add State(s) to Queue__jki_lib_state_machine.vi"("State(s) in (\"\")"=w415) -> ("States Out"=w414:string)  [unwired: 14 in]
          }
          frame "Events: Register" {
            w417 = T9 {"Error"=refnum, "State"=refnum, "Reserve State"=refnum}  # Listener Public Events
            # "Expand to add\nmore events"
            n146 = Unbundle By Name(w427) -> ("SMO"=w416:refnum<class "RemoteControl.lvclass">)
            n147 = call <vilib>:"GetProtectedEvents.vi"("SMO"=w416) -> ("error out"=w421:errorcluster, "SMO Protected Events"=w425:T10, "SMO out"=w419:refnum<class "RemoteControl.lvclass">)  [unwired: 8 in]
            n148 = call "RemoteControl.GetPrivateEvents.vi"("RemoteControl"=w419) -> ("error out"=w420:errorcluster, "RC Private Events"=w418:T11)  [unwired: 8 in, 1 out]
            n149 = register-events(w425, w418, w417) -> (reference out=w426:refnum<event-registration>, error out=w422:errorcluster)  [unwired: 2 in]
            n150 = Merge Errors(w420, w424, w422, w421) -> (w423:errorcluster)
            n151 = call <vilib>:"Add State(s) to Queue__jki_lib_state_machine.vi"("State(s) in (\"\")"=w429) -> ("States Out"=w428:string)  [unwired: 14 in]
          }
          frame "Events: Register Listener SMO" {
            w434 = T9 {"Error"=refnum, "State"=refnum, "Reserve State"=refnum}  # Listener Public Events
            n152 = Unbundle By Name(w441) -> ("Listener"=w435:refnum<class "RemoteControl.lvclass">)
            n153 = call <vilib>:"GetPublicEvents.vi"("SMO"=w435) -> ("error out"=w433:errorcluster, "Public Events"=w431:T9)  [unwired: 8 in, 1 out]
            n154 = Variant To Data(error in=w433, type=w434, Variant=w431) -> (data=w430:T9, error out=w432:errorcluster)
            n155 = register-events(reference=w436, w430) -> (reference out=w440:refnum<event-registration>, error out=w437:errorcluster)  [unwired: 3 in]
            n156 = Merge Errors(w439, w437, w432) -> (w438:errorcluster)
            n157 = call <vilib>:"Add State(s) to Queue__jki_lib_state_machine.vi"("State(s) in (\"\")"=w443) -> ("States Out"=w442:string)  [unwired: 14 in]
          }
          frame "Events: Unregister" {
            n158 = Unregister For Events(event registration refnum=w446, error in=w445) -> (error out=w444:errorcluster)
            n159 = call <vilib>:"Clear Errors.vi"("error in (no error)"=w444) -> ()  [unwired: 5 in, 2 out]
            n160 = call <vilib>:"Add State(s) to Queue__jki_lib_state_machine.vi"("State(s) in (\"\")"=w449) -> ("States Out"=w448:string)  [unwired: 14 in]
          }
          frame "---------- RC ----------" {
            # "Template Separator\n(You can make a copy of, or modify, this frame)"
            n161 = call <vilib>:"Add State(s) to Queue__jki_lib_state_machine.vi"("State(s) in (\"\")"=w454) -> ("States Out"=w453:string)  [unwired: 14 in]
          }
          frame "RC: Send Messages to Owner" {
            # "This loop will run # times equal to messages in the queue"
            # "Send Message to Owner to be processed\n(Send a message to the instrument to be processed)"
            n162 = Unbundle By Name(w455) -> ("SMO"=w459:refnum<class "RemoteControl.lvclass">, "Messages (in)"=w456:T3[])
            n163 = for {
              tunnel: w459 -> [w466]
              tunnel: w458 -> [w470]
              tunnel: w456 -> [w465] mode=indexing
              tunnel: w457 -> [w469]
              tunnel: [w464] -> w460
              n164 = call "Time Message Events.vi"("error in (no error)"=w469, "Debug Mode"=w470, "Message in"=w465, "RemoteControl"=w466) -> ("error out"=w471:errorcluster, "Message out"=w468:T3, "RemoteControl out"=w467:refnum<class "RemoteControl.lvclass">)  [unwired: 4 in, 1 out]
              n165 = call "RemoteControl.SendMessageFromProcess.vi"("error in (no error)"=w471, "Message"=w468, "RemoteControl"=w467) -> ("error out"=w464:errorcluster)  [unwired: 7 in, 1 out]
            }
            n166 = call <vilib>:"Add State(s) to Queue__jki_lib_state_machine.vi"("State(s) in (\"\")"=w463) -> ("States Out"=w462:string)  [unwired: 14 in]
          }
          frame "RC: Get Connections" {
            # "Here listen for new connections and then stop after timeout or if there's a new connection"
            n167 = Unbundle By Name(w478) -> ("SMO"=w477:refnum<class "RemoteControl.lvclass">)
            n168 = call-dynamic "Get Connections.vi"("error in (no error)"=w476, "RemoteControl in"=w477) -> ("error out"=w472:errorcluster, "Number"=w474:i32, "RemoteControl out"=w475:refnum<class "RemoteControl.lvclass">)  [unwired: 7 in]
            "Connections" <- w474
            n169 = case shown="Default" w474 {
              selector: w474 -> [_ w485 _]
              tunnel: ["" ("State(s) in Front (\"\")") w484 "RC: Close Connection" ("State(s) in Front (\"\")")] -> w473
              frame 0 {
              }
              frame Default {
                # "read %d messages"
                n170 = Format Into String(format string="RC: Read Messages >> %d" ("State(s) in Front (\"\")"), w485) -> (resulting string=w484:string)  [unwired: 2 in, 1 out]
              }
              frame 100 {
              }
            }
            n171 = Bundle By Name(cluster=w478, "SMO"=w475) -> (w479:T6)
            n172 = call <vilib>:"Add State(s) to Queue__jki_lib_state_machine.vi"("State(s) in Front (\"\")"=w473, "State(s) in (\"\")"=w482) -> ("States Out"=w481:string)  [unwired: 13 in]
          }
          frame "RC: Read Messages" {
            # "poll the number\nof open connections"
            # "Read Message over, eg TCP"
            # "If command is empty do not Send Message"
            n173 = Unbundle By Name(w497) -> ("to"=w500:i32)
            n174 = Unbundle By Name(w497) -> ("SMO"=w496:refnum<class "RemoteControl.lvclass">)
            n175 = call "Write Timeout.vi"("error in (no error)"=w495, "timeout (ms) [500]"="timeout (ms)", "RemoteControl in"=w496) -> ("error out"=w494:errorcluster, "RemoteControl out"=w493:refnum<class "RemoteControl.lvclass">)  [unwired: 7 in]
            n176 = call-dynamic "Read Message.vi"("error in (no error)"=w494, "RemoteControl in"=w493) -> ("error out"=w499:errorcluster, "Message"=w489:T3, "RemoteControl out"=w498:refnum<class "RemoteControl.lvclass">)  [unwired: 7 in]
            n177 = Unbundle By Name(w489) -> ("Command"=w488:string)
            n178 = case shown="Default" w488 {
              tunnel: w499 -> [w514 w524]
              tunnel: [w514 w524] -> w502
              tunnel: w506 -> [_ _]
              tunnel: w498 -> [w513 w519]
              tunnel: [enum16{"waiting", "processing"}."processing" ("state") enum16{"waiting", "processing"}."waiting" ("state")] -> w504
              tunnel: ["RC: Send Messages to Owner" ""] -> w503
              tunnel: [5000 w523] -> w501
              tunnel: w500 -> [_ w523]
              tunnel: [w511 w520] -> w491
              tunnel: [w513 w519] -> w490
              tunnel: w489 -> [w510 _]
              frame Default {
                n179 = Build Array(w510) -> (w511:T3[])
                n180 = call "Message to Display String.vi"("Message"=w510) -> ("message string"=→"Message In":string)
              }
              frame "" {
                # "Messages coming from TCP need to have command"
                n181 = Build Array(T3 {"Command"="", "Data"=variant(string ""), "ID"="", "error"={"status"=FALSE, "code"=0, "source"=""}} ("Message out")) -> (w520:T3[])
              }
            }
            n182 = Bundle By Name(cluster=w497, "to"=w501, "state"=w504, "SMO"=w490, "Messages (in)"=w491) -> (w505:T6)
            n183 = call <vilib>:"Add State(s) to Queue__jki_lib_state_machine.vi"("State(s) in Front (\"\")"=w503, "State(s) in (\"\")"=w509) -> ("States Out"=w508:string)  [unwired: 13 in]
          }
          frame "RC: Write Messages" {
            # "After the loop completes\nempty the out queue"
            # "This loop will run # times equal to messages in the out queue"
            # "send Message over, eg. TCP"
            n184 = Unbundle By Name(w530) -> ("SMO"=w535:refnum<class "RemoteControl.lvclass">, "Messages (out)"=w533:T3[])
            n185 = for {
              tunnel: w535 -> [w541]
              tunnel: w534 -> [w540]
              tunnel: w533 -> [w544] mode=indexing
              tunnel: [w545] -> w525
              tunnel: w532 -> [w548]
              tunnel: [w539] -> w531
              n186 = call "Time Message Events.vi"("error in (no error)"=w548, "Debug Mode"=w540, "Message in"=w544, "RemoteControl"=w541) -> ("error out"=w547:errorcluster, "Message out"=w543:T3, "RemoteControl out"=w542:refnum<class "RemoteControl.lvclass">)  [unwired: 4 in, 1 out]
              n187 = while {
                tunnel: w547 -> [w550]
                tunnel: [w550] -> w546
                stop <- "delay response" continue-if-true
              }
              n188 = call-dynamic "Send Message.vi"("error in (no error)"=w546, "Message"=w543, "RemoteControl in"=w542) -> ("error out"=w539:errorcluster, "RemoteControl out"=w545:refnum<class "RemoteControl.lvclass">)  [unwired: 7 in]
            }
            n189 = Bundle By Name(cluster=w530, "Messages (out)"=T3[] [], "state"=enum16{"waiting", "processing"}."waiting", "to"=5, "SMO"=w525) -> (w529:T6)
            n190 = call <vilib>:"Add State(s) to Queue__jki_lib_state_machine.vi"("State(s) in (\"\")"=w538) -> ("States Out"=w537:string)  [unwired: 14 in]
          }
          frame "RC: Close Connection" {
            # "Closes open server connections"
            # "call this on error 66, etc (when connection\ndrops). check these in error handler"
            n191 = Unbundle By Name(w555) -> ("SMO"=w556:refnum<class "RemoteControl.lvclass">)
            n192 = call-dynamic "Close Connection.vi"("error in (no error)"=w552, "RemoteControl in"=w556) -> ("error out"=w551:errorcluster, "RemoteControl out"=w553:refnum<class "RemoteControl.lvclass">)  [unwired: 8 in]
            n193 = Bundle By Name(cluster=w555, "SMO"=w553) -> (w554:T6)
            n194 = call <vilib>:"Add State(s) to Queue__jki_lib_state_machine.vi"("State(s) in (\"\")"=w559) -> ("States Out"=w558:string)  [unwired: 14 in]
          }
          frame "RC: Create Listener SMO" {
            # "Create Listener SMO"
            n195 = Unbundle By Name(w569) -> ("SMO"=w562:refnum<class "RemoteControl.lvclass">, "Configure"=w564:T5)
            n196 = Bundle By Name(cluster=w562, "Configure"=w564, "RC Process Type"=RC_Process_Type--Enum."Listener") -> (w561:refnum<class "RemoteControl.lvclass">)
            n197 = call <vilib>:"Create.vi"("error in (no error)"=w560, "Subsystem Name (optional)"="Remote-Control-Listener" ("format string"), "SMO"=w561) -> ("error out"=w567:errorcluster, "SMO out"=w563:refnum<class "RemoteControl.lvclass">)  [unwired: 6 in, 1 out]
            n198 = Bundle By Name(cluster=w569, "Listener"=w563) -> (w568:T6)
            n199 = call <vilib>:"Add State(s) to Queue__jki_lib_state_machine.vi"("State(s) in (\"\")"=w572) -> ("States Out"=w571:string)  [unwired: 14 in]
          }
          frame "RC: Start Listener SMO" {
            n200 = Unbundle By Name(w578) -> ("Listener"=w575:refnum<class "RemoteControl.lvclass">)
            n201 = call <vilib>:"Start.vi"("error in (no error)"=w574, "SMO"=w575) -> ("error out"=w573:errorcluster, "SMO out"=w576:refnum<class "RemoteControl.lvclass">)  [unwired: 8 in]
            n202 = Bundle By Name(cluster=w578, "Listener"=w576) -> (w577:T6)
            n203 = call <vilib>:"Add State(s) to Queue__jki_lib_state_machine.vi"("State(s) in (\"\")"=w581) -> ("States Out"=w580:string)  [unwired: 14 in]
          }
          frame "RC: Stop Listener SMO" {
            n204 = Unbundle By Name(w585) -> ("Listener"=w586:refnum<class "RemoteControl.lvclass">)
            n205 = call <vilib>:"Stop.vi"("error in (no error)"=w583, "SMO"=w586) -> ("error out"=w582:errorcluster, "SMO out"=w587:refnum<class "RemoteControl.lvclass">)  [unwired: 8 in]
            n206 = Bundle By Name(cluster=w585, "Listener"=w587) -> (w584:T6)
            n207 = call <vilib>:"Add State(s) to Queue__jki_lib_state_machine.vi"("State(s) in (\"\")"=w590) -> ("States Out"=w589:string)  [unwired: 14 in]
          }
          frame "RC: Destroy Listener SMO" {
            n208 = Unbundle By Name(w592) -> ("Listener"=w593:refnum<class "RemoteControl.lvclass">)
            n209 = call <vilib>:"Destroy.vi"("error in (no error)"=w594, "SMO"=w593) -> ("error out"=w591:errorcluster)  [unwired: 9 in]
            n210 = call <vilib>:"Add State(s) to Queue__jki_lib_state_machine.vi"("State(s) in (\"\")"=w597) -> ("States Out"=w596:string)  [unwired: 14 in]
          }
          frame "RC: Open Client Connection" {
            n211 = Unbundle By Name(w601) -> ("SMO"=w605:refnum<class "RemoteControl.lvclass">, "Configure.address"=w599:string, "Configure.Port"=w598:u16)
            n212 = call-dynamic "Open Client Connection.vi"("error in (no error)"=w604, "Port"=w598, "address"=w599, "RemoteControl in"=w605) -> ("error out"=w603:errorcluster, "RemoteControl out"=w602:refnum<class "RemoteControl.lvclass">)  [unwired: 6 in]
            n213 = Bundle By Name(cluster=w601, "SMO"=w602) -> (w600:T6)
            n214 = call <vilib>:"Add State(s) to Queue__jki_lib_state_machine.vi"("State(s) in (\"\")"=w608) -> ("States Out"=w607:string)  [unwired: 14 in]
          }
          frame "RC: Open Server Connection" {
            n215 = Unbundle By Name(w609) -> ("SMO"=w616:refnum<class "RemoteControl.lvclass">, "Configure.address"=w611:string, "Configure.Port"=w610:u16)
            n216 = call-dynamic "Open Server Connection.vi"("error in (no error)"=w615, "Port"=w610, "address"=w611, "RemoteControl in"=w616) -> ("error out"=w614:errorcluster, "RemoteControl out"=w613:refnum<class "RemoteControl.lvclass">)  [unwired: 6 in]
            n217 = Bundle By Name(cluster=w609, "SMO"=w613) -> (w612:T6)
            n218 = call <vilib>:"Add State(s) to Queue__jki_lib_state_machine.vi"("State(s) in (\"\")"=w619) -> ("States Out"=w618:string)  [unwired: 14 in]
          }
          frame "---------- Listener ----------" {
            # "Template Separator\n(You can make a copy of, or modify, this frame)"
            n219 = call <vilib>:"Add State(s) to Queue__jki_lib_state_machine.vi"("State(s) in (\"\")"=w624) -> ("States Out"=w623:string)  [unwired: 14 in]
          }
          frame "Listener: Start Listener" {
            # "Start Asynchronous Listener"
            n220 = Unbundle By Name(w625) -> ("SMO"=w630:refnum<class "RemoteControl.lvclass">)
            n221 = call-dynamic "Start Listener.vi"("error in (no error)"=w629, "RemoteControl in"=w630) -> ("error out"=w628:errorcluster, "RemoteControl out"=w627:refnum<class "RemoteControl.lvclass">)  [unwired: 8 in]
            n222 = Bundle By Name(cluster=w625, "SMO"=w627) -> (w626:T6)
            n223 = call <vilib>:"Add State(s) to Queue__jki_lib_state_machine.vi"("State(s) in (\"\")"=w633) -> ("States Out"=w632:string)  [unwired: 14 in]
          }
          frame "Listener: Listen" {
            n224 = Unbundle By Name(w642) -> ("SMO"=w639:refnum<class "RemoteControl.lvclass">)
            n225 = call-dynamic "Listen.vi"("timeout ms (100) (wait forever: -1)"=1000, "error in (no error)"=w638, "RemoteControl"=w639) -> ("error out"=w635:errorcluster, "RemoteControl out"=w640:refnum<class "RemoteControl.lvclass">)  [unwired: 7 in]
            n226 = case shown="True" "create listener error" {
              tunnel: w635 -> [w646 _]
              tunnel: [w646 errorcluster {"status"=TRUE, "code"=-1000, "source"="Listener error"} ("t")] -> w634
              frame False {
              }
              frame True {
                n227 = local write "create listener error"(FALSE ("create listener error")) -> ()
              }
            }
            n228 = Bundle By Name(cluster=w642, "SMO"=w640) -> (w641:T6)
            n229 = call <vilib>:"Add State(s) to Queue__jki_lib_state_machine.vi"("State(s) in (\"\")"=w645) -> ("States Out"=w644:string)  [unwired: 14 in]
          }
          frame "Listener: Stop Listener" {
            # "Stop Asynchronous Listener \n(You can make a copy of, or modify, this frame)"
            n230 = Unbundle By Name(w649) -> ("SMO"=w652:refnum<class "RemoteControl.lvclass">)
            n231 = call-dynamic "Stop Listener.vi"("error in (no error)"=w651, "RemoteControl in"=w652) -> ("error out"=w650:errorcluster)  [unwired: 8 in, 1 out]
            n232 = call <vilib>:"Add State(s) to Queue__jki_lib_state_machine.vi"("State(s) in (\"\")"=w655) -> ("States Out"=w654:string)  [unwired: 14 in]
          }
        }
      }
    }
    frame Error {
    }
  }
  n233 = call-parent "Process.vi"("error in"=w3, "SMO"=w2) -> ("error out"=w1:errorcluster, "SMO out"=→"RemoteControl out":refnum<class "RemoteControl.lvclass">)  [unwired: 8 in]
  n234 = Merge Errors(w1, w5) -> (→"error out":errorcluster)
